vi "RL Custom Data.vi"() -> (7 "custom output":string)   [LabVIEW 2014]
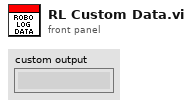
[diagram p1: front panel]
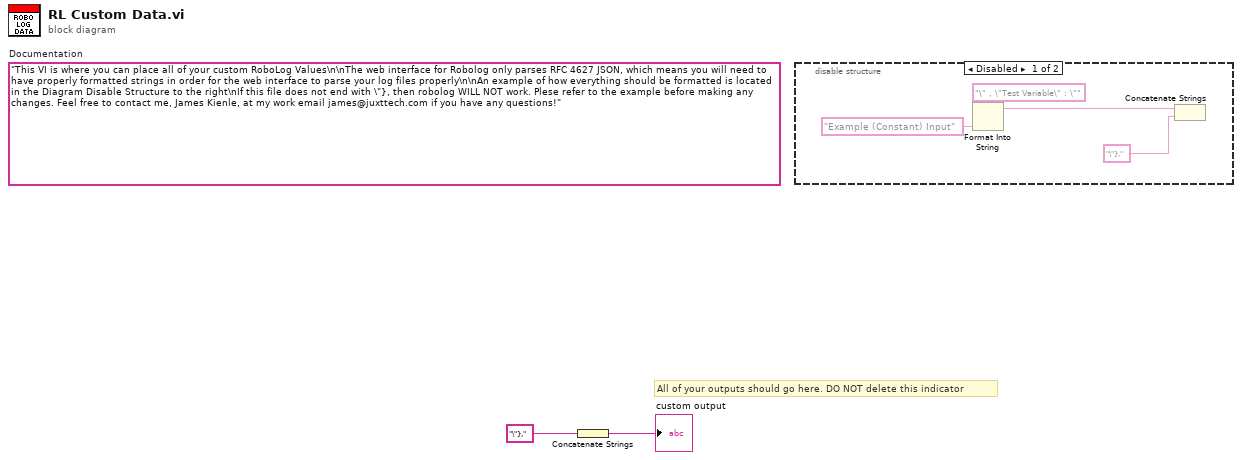
[diagram p0: block diagram]
diagram:
  (unwired) "This VI is where you can place all of your custom RoboLog Values\n\nThe web interface for Robolog only parses RFC 4627 JSON, which means you will need to have properly formatted strings in order for the web interface to parse your log files properly\n\nAn example of how everything should be formatted is located in the Diagram Disable Structure to the right\nIf this file does not end with \"}, then robolog WILL NOT work. Plese refer to the example before making any changes. Feel free to contact me, James Kienle, at my work email james@juxttech.com if you have any questions!"  # Documentation
  # "All of your outputs should go here. DO NOT delete this indicator"
  n1 = Concatenate Strings("\"}," ("string")) -> (→"custom output":string)
  n2 = disable-structure shown="Disabled" {
    frame Disabled {
      n3 = Format Into String(initial string="\" , \"Test Variable\" : \"", "Example (Constant) Input" ("input 1")) -> (resulting string=w4:string)  [unwired: 2 in, 1 out]
      n4 = Concatenate Strings(w4, "\"}," ("string")) -> ()  [unwired: 1 out]
    }
    frame Enabled {
    }
  }
